vi "File Viewer (2).vi"() -> ()   [LabVIEW 2018]
uses:
  <vilib>/Utility/file.llb/Read Delimited Spreadsheet (I64).vi
  <vilib>/Utility/file.llb/Write Delimited Spreadsheet (I64).vi
panel:
  in  "file path (dialog if empty)":path
  out "Waveform Graph":i64[](graph)
  in  "Numeric":dbl
  in  "file path for picture":path
  in  "?":bool
  out "Intensity Graph":i64[][](graph)
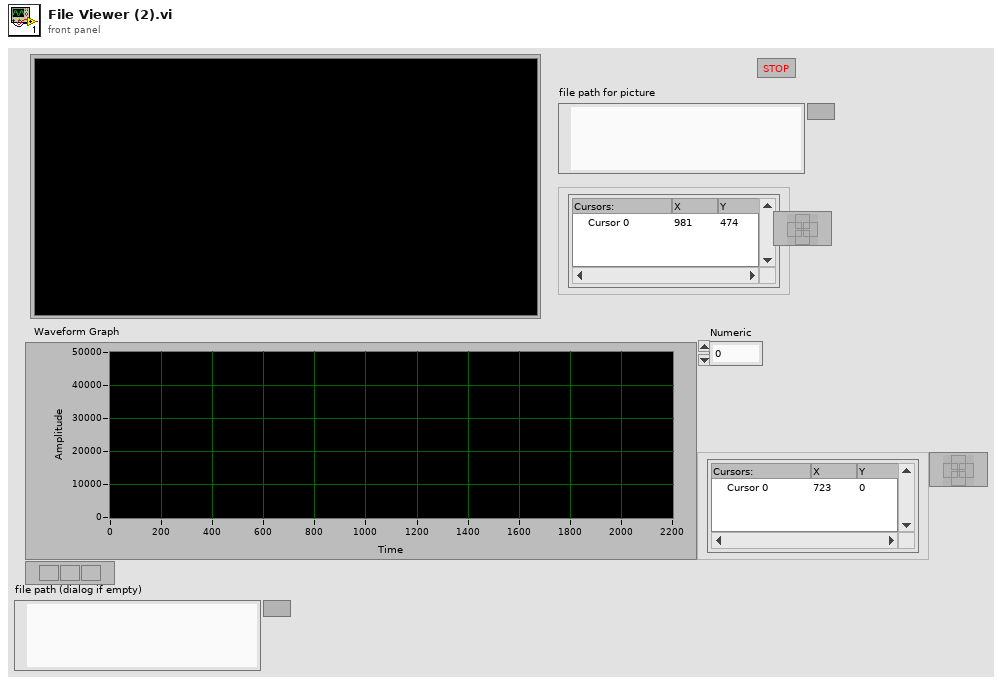
[diagram p1: front panel]
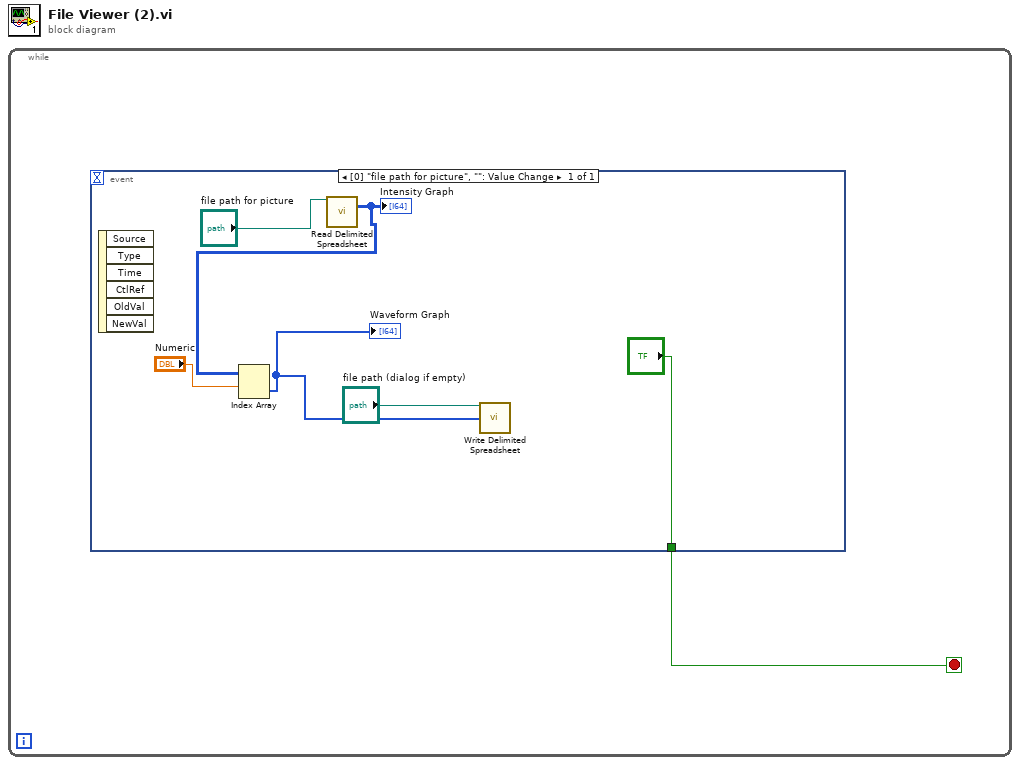
[diagram p0: block diagram]
diagram:
  n1 = while {
    stop <- w1 stop-if-true
    n2 = event shown="[0] \"file path for picture\", \"\": Value Change" {
      selector: _ -> [_]
      dyn-events: _ -> [_]
      timeout: _ -> [_]
      tunnel: ["?"] -> w1
      event "file path for picture": Value Change {
        n3 = event-data() -> ()  [unwired: 1 in, 6 out]
        n4 = call-poly <vilib>:"Read Delimited Spreadsheet.vi"("file path (dialog if empty)"="file path for picture") -> ("all rows"=w7:i64[][])  [unwired: 9 in, 5 out]
        "Intensity Graph" <- w7
        n5 = Index Array(array=w7, index (row)="Numeric") -> (element=w3:i64[])  [unwired: 1 in]
        "Waveform Graph" <- w3
        n6 = call-poly <vilib>:"Write Delimited Spreadsheet.vi"("file path (dialog if empty)"="file path (dialog if empty)", "1D data"=w3) -> ()  [unwired: 12 in, 2 out]
      }
    }
  }
